vi "Simulation Noninteractive Run.vi"(11 "simulation configuration":T2={"maxTime"=inf, "enableVisualization"=TRUE, "Environment Definition"=path "Environment - Navigation and Hill Climb 1.xml", "Record Location"=path "Simulation Record.xml", "autograde?"=TRUE, "interactive?"=FALSE, "Feedback Mode"=enum."debug navigation", "Robot State Charts"=[path "C:/Users/blueuser/Desktop/Robo Sim Berkley/cpsgrader-release-0.4/Simulators/EECS149lab/src/LabVIEW/statechart/Simulation Statechart.vi"], "statechart"=path "Simulation Statechart.vi"}) -> (0 "error out":errorcluster, 3 "record":T1={"configuration"={"maxTime"=5.0, "enableVisualization"=TRUE, "Environment Definition"=path "iRobot Navigation State Machine.vi", "Record Location"=path "Simulation Record.xml", "autograde?"=TRUE, "interactive?"=FALSE, "Feedback Mode"=enum."debug navigation", "Robot State Charts"=[path "C:/Users/blueuser/Desktop/Robo Sim Berkley/cpsgrader-release-0.4/Simulators/EECS149lab/src/LabVIEW/statechart/Simulation Statechart.vi"], "statechart"=path "iRobot Navigation State Machine.vi"}, "trace"=[], "environment MD5"="", "statechart MD5"="", "record timestamp"=""} {"trace"."sensors"."accelerometer"."z axis (g)" format="%.3f"; "trace"."sensors"."accelerometer"."y axis (g)" format="%.3f"; "trace"."sensors"."accelerometer"."x axis (g)" format="%.3f"})   [LabVIEW 2014]
uses:
  Simulation Call Statechart Operation.ctl
  CyberSim interface/Simulation Configuration.ctl
  shared/Accelerometer.ctl
  Kobuki/Charging Sources Available.ctl
  shared/Sensors.ctl
  Simulated Position.ctl
  Simulated Orientation.ctl
  Simulation Trace Element.ctl
  Simulation Record.ctl
  autograder/feedbackMode.ctl
  Kobuki/Kobuki Bumps and WheelDrops.ctl
  Kobuki/Kobuki Buttons.ctl
  Kobuki/KobukiSensors.ctl
panel:
  # "Electrical: charging, battery, OI mode"
  # "Sensors: bump, cliff, button, wheel drop, wall, virtual wall"
  # "Motors:"
  # "Song"
  # "Inertia"
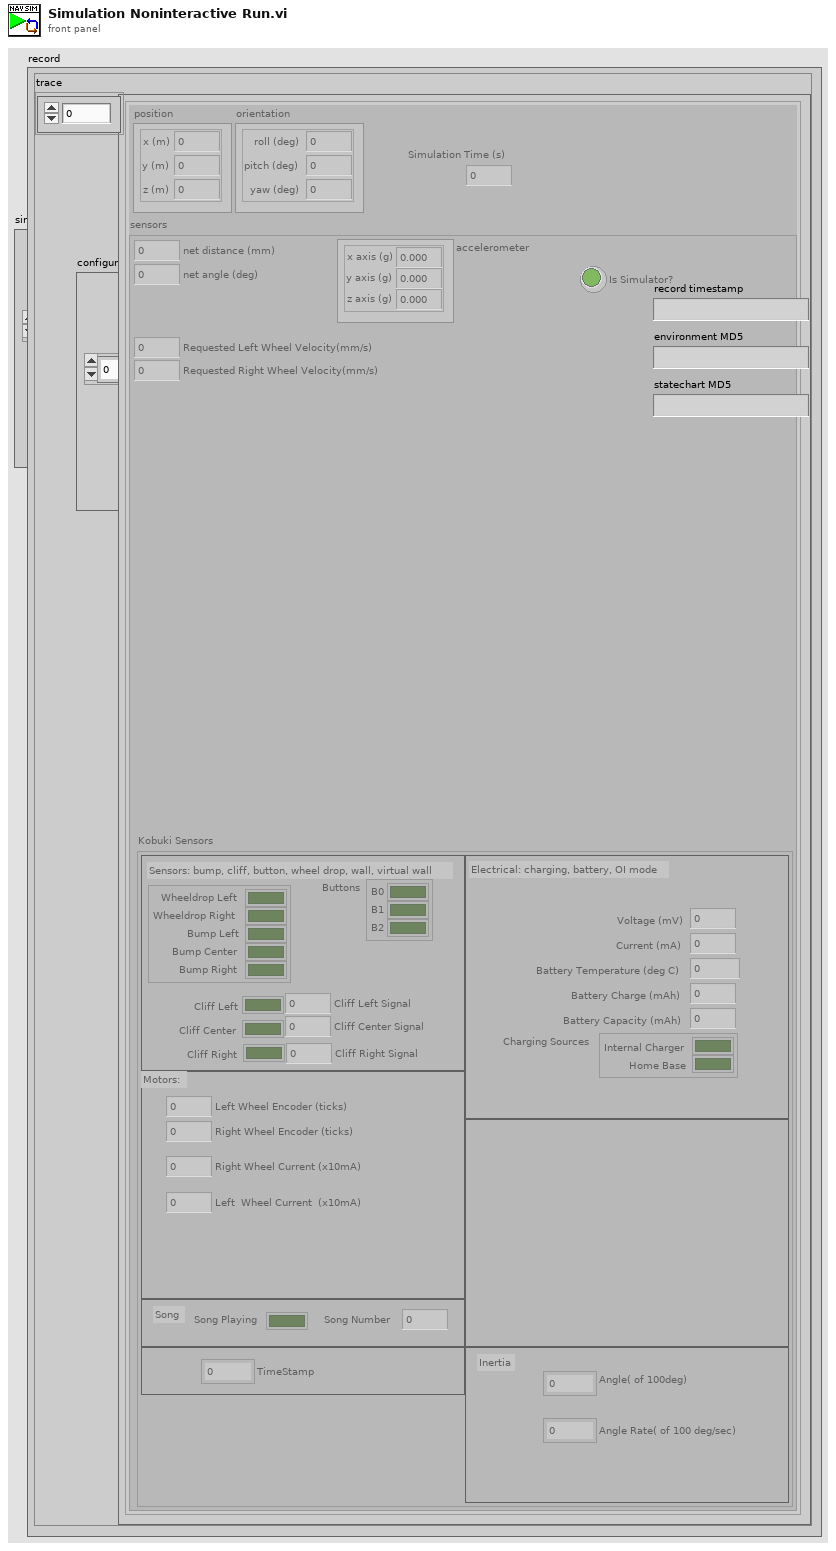
[diagram p1: front panel]
types:
  T1 = typedef "Simulation Record.ctl" = cluster{"configuration":T2, "trace":T4[], "environment MD5":string, "statechart MD5":string, "record timestamp":string}
  T2 = typedef "Simulation Configuration.ctl" = cluster{"maxTime":sgl, "enableVisualization":bool, "Environment Definition":path, "Record Location":path, "autograde?":bool, "interactive?":bool, "Feedback Mode":T3, "Robot State Charts":path[], "statechart":path}
  T3 = typedef "feedbackMode.ctl" = enum32{"debug navigation", "debug hill climb", "autograde navigation", "autograde hill climb"}
  T4 = typedef "Simulation Trace Element.ctl" = cluster{"sensors":T5, "position":T11, "orientation":T12, "Simulation Time (s)":sgl}
  T5 = typedef "Sensors.ctl" = cluster{"net distance (mm)":i32, "net angle (deg)":i32, "accelerometer":T6, "Is Simulator?":bool, "Kobuki Sensors":T7, "Requested Left Wheel Velocity(mm/s)":i32, "Requested Right Wheel Velocity(mm/s)":i32}
  T6 = typedef "Accelerometer.ctl" = cluster{"x axis (g)":dbl, "y axis (g)":dbl, "z axis (g)":dbl}
  T7 = typedef "KobukiSensors.ctl" = cluster{"Bumps + Wheel Drops":T8, "Cliff Left":bool, "Cliff Center":bool, "Cliff Right":bool, "Cliff Left Signal":u16, "Cliff Center Signal":u16, "Cliff Right Signal":u16, "Buttons":T9, "Left Wheel Encoder (ticks)":u16, "Right Wheel Encoder (ticks) ":u16, "Right Wheel Current (x10mA)":i16, "Left  Wheel Current  (x10mA)":i16, "TimeStamp":u16, "Song Playing":bool, "Song Number":u8, "Voltage (mV)":i16, "Current (mA)":i16, "Battery Temperature (deg C)":i16, "Battery Charge (mAh)":i16, "Battery Capacity (mAh)":i16, "Charging Sources":T10, "Angle( of 100deg)":i16, "Angle Rate( of 100 deg/sec)":i16}
  T8 = typedef "Kobuki Bumps and WheelDrops.ctl" = cluster{"Wheeldrop Left":bool, "Wheeldrop Right":bool, "Bump Left":bool, "Bump Center":bool, "Bump Right":bool}
  T9 = typedef "Kobuki Buttons.ctl" = cluster{"B0":bool, "B1":bool, "B2":bool}
  T10 = typedef "Charging Sources Available.ctl" = cluster{"Internal Charger":bool, "Home Base":bool}
  T11 = typedef "Simulated Position.ctl" = cluster{"x (m)":sgl, "y (m)":sgl, "z (m)":sgl}
  T12 = typedef "Simulated Orientation.ctl" = cluster{"roll (deg)":sgl, "pitch (deg)":sgl, "yaw (deg)":sgl}
  T13 = typedef "Simulation Call Statechart Operation.ctl" = enum16{"Initialize", "Call Statechart", "Finalize"}
  T14 = typedef "Simulator.ctl" = cluster{"configuration":T2, "Statechart\ndisplay":refnum<vi>, "first step?":bool, "Robots Simulation Statecharts":path[], "Robots":T15[]}
  T15 = typedef "RobotData.ctl" = cluster{"Bump Sensors":refnum<k20>[], "Distance Sensors":refnum<k20>[], "Accelerometer":refnum<k20>, "Wall Sensor":refnum<k20>, "Body":refnum<k20>, "RobotID":string, "RobotType":string, "Left Motor":refnum<class "DC Motor Controller.lvclass">, "Right Motor":refnum<class "DC Motor Controller.lvclass">}
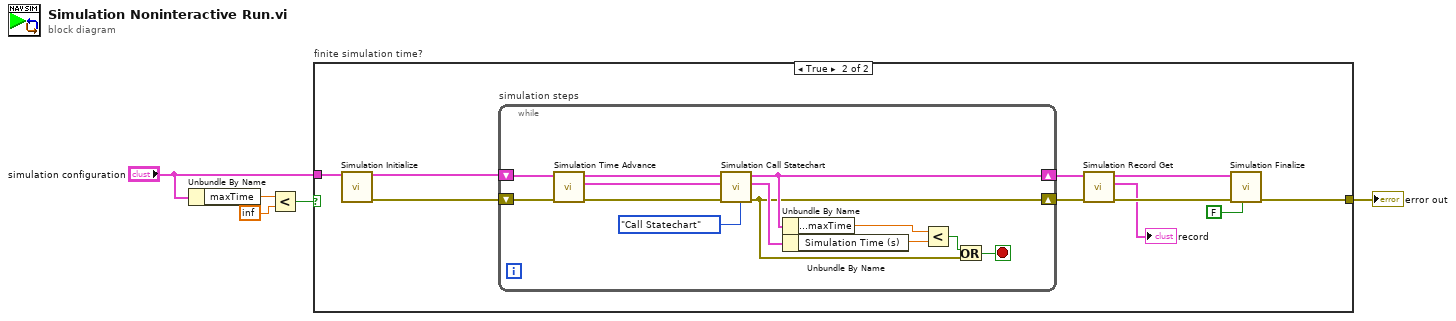
[diagram p0: block diagram]
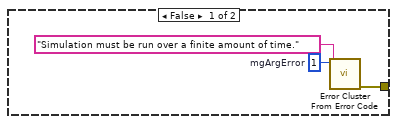
[diagram p2: hidden frame]
diagram:
  n1 = Unbundle By Name("simulation configuration") -> ("maxTime"=w3:sgl)
  n2 = Less?(x=w3, y=sgl inf) -> (x < y?=w1:bool)
  n3 = case "finite simulation time?" shown="True" w1 {
    tunnel: [w8 w16] -> w5
    tunnel: "simulation configuration" -> [_ w15]
    frame False {
      w7 = 1  # mgArgError
      n4 = call <vilib>:"Error Cluster From Error Code.vi"("error message (\"\")"="Simulation must be run over a finite amount of time." ("error message (\"\")"), "error code (0)"=w7) -> ("error out"=w8:errorcluster)  [unwired: 7 in]
    }
    frame True {
      n5 = call "Simulation Initialize.vi"("simulation configuration"=w15) -> ("simulator"=w18:T14, "Error Out"=w17:errorcluster)  [unwired: 13 in]
      n6 = while "simulation steps" {
        shift-right: [w20] -> w14
        shift-left: w18 -> [w27]
        shift-right: [w19] -> w13
        shift-left: w17 -> [w26]
        stop <- w21 stop-if-true
        n7 = call "Simulation Time Advance.vi"("error in (no error)"=w26, "simulator"=w27) -> ("error out"=w29:errorcluster, "Robot Sensors"=w30:T5[], "simulator"=w31:T14)  [unwired: 7 in]
        n8 = call "Simulation Call Statechart.vi"("operation"=Simulation_Call_Statechart_Operation."Call Statechart", "error in"=w29, "Multi Bot Sensors"=w30, "simulator"=w31) -> ("error out"=w19:errorcluster, "trace element"=w23:T4, "simulator"=w20:T14)  [unwired: 5 in]
        n9 = Unbundle By Name(w20) -> ("configuration.maxTime"=w25:sgl)
        n10 = Unbundle By Name(w23) -> ("Simulation Time (s)"=w24:sgl)
        n11 = Less?(x=w25, y=w24) -> (x < y?=w22:bool)
        n12 = Or(x=w22, y=w19) -> (x .or. y?=w21:bool)
      }
      n13 = call "Simulation Record Get.vi"("Error In"=w13, "simulator"=w14) -> ("Error Out"=w11:errorcluster, "record"=→"record":T1, "simulator"=w12:T14)  [unwired: 7 in]
      n14 = call "Simulation Finalize.vi"("terminated by user?"=FALSE, "error in (no error)"=w11, "simulator"=w12) -> ("error out"=w16:errorcluster)  [unwired: 7 in, 1 out]
    }
  }
  "error out" <- w5
